vi "SSC Digital Configure Termination Mode.vi"(0 "Digital SSC in":T1[](array[typedef]), 5 "Termination Mode":T2=1202 items=["High Z"=1202, "Active Load"=1200, "Vterm"=1201], 11 "error in":errorcluster) -> (4 "Digital SSC out":T1[](array[typedef]), 15 "error out":errorcluster)   [LabVIEW 2020]
doc: "Specifies the behavior of the specified pin(s) and pin group(s) when the pin driver is in a non-drive pin state (L, H, X, V, M, E)."
uses:
  <instrlib>/niDigital/niDigital.llb/niDigital Termination Mode.ctl
  SSC Digital.ctl
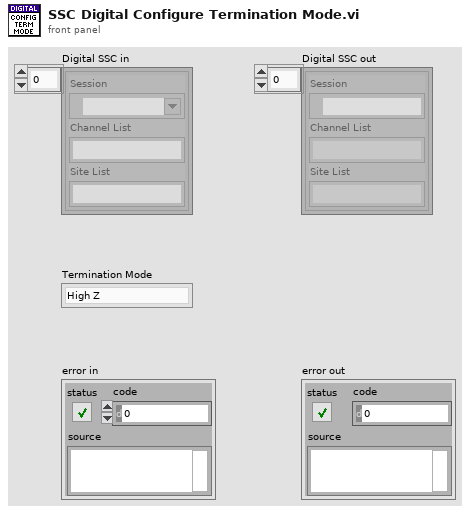
[diagram p1: front panel]
types:
  T1 = typedef "SSC Digital.ctl" = cluster{"Session":refnum<k15>, "Channel List":string, "Site List":string}
  T2 = typedef "niDigital Termination Mode.ctl" = i32
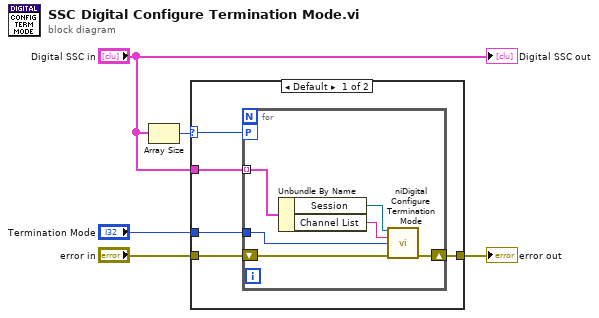
[diagram p0: block diagram]
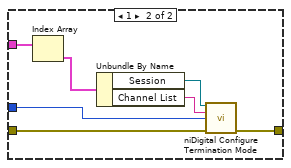
[diagram p2: hidden frame]
diagram:
  n1 = Array Size(array="Digital SSC in") -> (size(s)=w2:i32)
  n2 = case shown="Default" w2 {
    selector: w2 -> [w7 _]
    tunnel: "error in" -> [w10 w23]
    tunnel: "Termination Mode" -> [w9 w22]
    tunnel: [w8 w21] -> w3
    tunnel: "Digital SSC in" -> [w6 w20]
    frame Default {
      n3 = for {
        workers-P: w7 -> [_]
        tunnel: w9 -> [w14]
        tunnel: w6 -> [w13] mode=indexing
        shift-right: [w15] -> w8
        shift-left: w10 -> [w16]
        n4 = Unbundle By Name(w13) -> ("Session"=w12:refnum<k15>, "Channel List"=w11:string)
        n5 = call <instrlib>:"niDigital Configure Termination Mode.vi"("instrument handle"=w12, "channel list"=w11, "termination mode"=w14, "error in"=w16) -> ("error out"=w15:errorcluster)  [unwired: 10 in, 1 out]
      }
    }
    frame 1 {
      n6 = Index Array(array=w20) -> (element=w17:T1)  [unwired: 1 in]
      n7 = Unbundle By Name(w17) -> ("Session"=w19:refnum<k15>, "Channel List"=w18:string)
      n8 = call <instrlib>:"niDigital Configure Termination Mode.vi"("instrument handle"=w19, "channel list"=w18, "termination mode"=w22, "error in"=w23) -> ("error out"=w21:errorcluster)  [unwired: 10 in, 1 out]
    }
  }
  "error out" <- w3
  "Digital SSC out" <- "Digital SSC in"
